vi "MC5e Check Unit is Unique.vi"(6 "index":i32, 7 "Mode":T7, 10 "Unit":T1={"Unit Fatigue Level"=enum."Not Fatigued", "Flying Unit"=FALSE, "Mounted Unit"=FALSE, "Defending from Stronghold"=FALSE, "Difficult Terrain Types"=[0, 1, 3, 6, 7], "Squads in Unit"=[], "Unit Info"={"Unit Name"="", "Unit Commander"="", "Morale Mod"=0, "BR Mod"=0, "Defense Mod"=0, "Speed Mod"=0, "Unit Notes"="", "Attack Mod"=0, "Unit Wins+ Losses-"=0, "Commander Charisma Bonus"=0}, "Range"=0, "BR"=0, "Speed"=0, "Morale"=0, "Current BR"=0, "Location"={"X coordinate"=0.0, "Y coordinate"=0.0}, "Capacity %"=0} {"Squads in Unit"."CR" items=["30", "29", "28", "27", "26", "25", "24", "23", "22", "21", "20", "19", "18", "17", "16", "15", "14", "13", "12", "11", "10", "9", "8", "7", "6", "5", "4", "3", "2", "1", "1/2", "1/4", "1/8"]}) -> (1 "Unit Name is Valid":bool, 2 "Unit Out (Duplicate)":T1={"Unit Fatigue Level"=enum."Not Fatigued", "Flying Unit"=FALSE, "Mounted Unit"=FALSE, "Defending from Stronghold"=FALSE, "Difficult Terrain Types"=[0, 1, 3, 6, 7], "Squads in Unit"=[], "Unit Info"={"Unit Name"="", "Unit Commander"="", "Morale Mod"=0, "BR Mod"=0, "Defense Mod"=0, "Speed Mod"=0, "Unit Notes"="", "Attack Mod"=0, "Unit Wins+ Losses-"=0, "Commander Charisma Bonus"=0}, "Range"=0, "BR"=0, "Speed"=0, "Morale"=0, "Current BR"=0, "Location"={"X coordinate"=0.0, "Y coordinate"=0.0}, "Capacity %"=0} {"Squads in Unit"."CR" items=["30", "29", "28", "27", "26", "25", "24", "23", "22", "21", "20", "19", "18", "17", "16", "15", "14", "13", "12", "11", "10", "9", "8", "7", "6", "5", "4", "3", "2", "1", "1/2", "1/4", "1/8"]}, 3 "OK Button Disabled?":T8(ring))   [LabVIEW 2020]
uses:
  MC5e Editor modes.ctl
  MC5e Unit.ctl
  MC5e Terrain types.ctl
  MC5e Squad_Info.ctl
  MC5e Size_Categories.ctl
  MC5e Unit Header.ctl
  Location.ctl
panel:
  # "Squads are restricted to one type of soldier (i.e  Archers) and all of the same level.\nIf you want mixed CR or mixed types, use multiple squads."
  # "Squads are restricted to one type of soldier (i.e  Archers) and all of the same level.\nIf you want mixed CR or mixed types, use multiple squads."
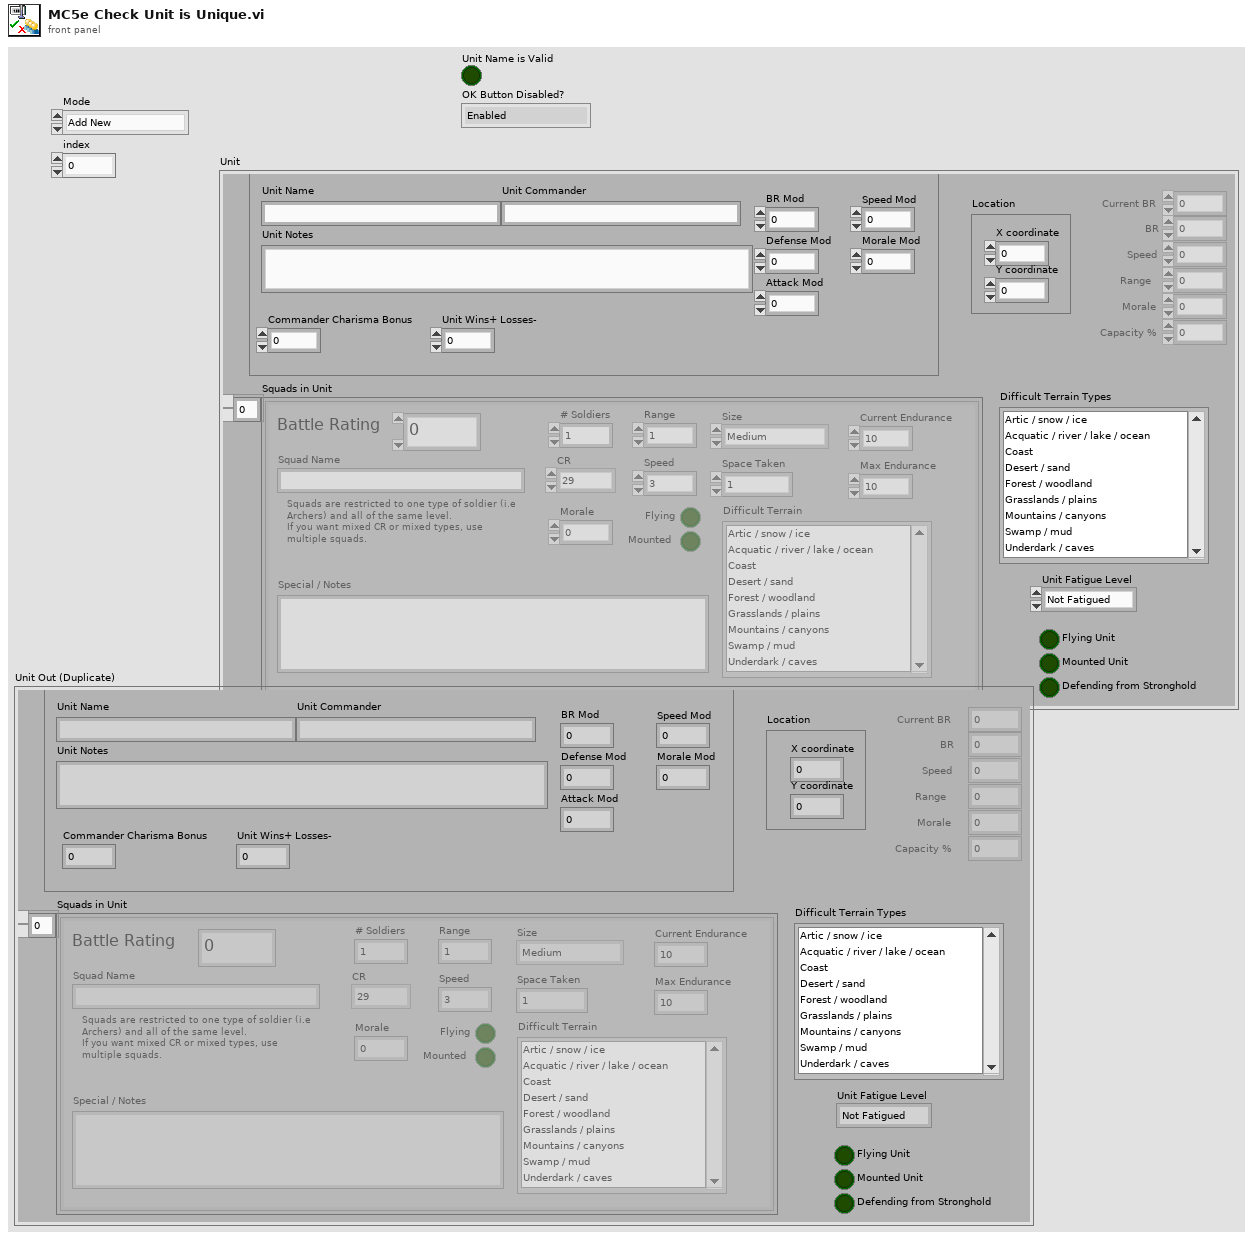
[diagram p1: front panel]
types:
  T1 = typedef "MC5e Unit.ctl" = cluster{"Unit Fatigue Level":enum16{"Not Fatigued", "Fatigued", "Seriously Fatigued"}, "Flying Unit":bool, "Mounted Unit":bool, "Defending from Stronghold":bool, "Difficult Terrain Types":T2, "Squads in Unit":T3[], "Unit Info":T5, "Range":i32, "BR":i32, "Speed":i32, "Morale":i32, "Current BR":i32, "Location":T6, "Capacity %":i32}
  T2 = typedef "MC5e Terrain types.ctl" = i32[]
  T3 = typedef "MC5e Squad_Info.ctl" = cluster{"Squad Name":string, "# Soldiers":u16, "Battle Rating":u16, "Flying":bool, "Mounted":bool, "Speed":u16, "Range":u16, "Morale":i32, "Max Endurance":u16, "Current Endurance":i32, "Size":T4, "Space Taken":u16, "Difficult Terrain":i32[], "CR":u16, "Special / Notes":string}
  T4 = typedef "MC5e Size_Categories.ctl" = enum16{"Tiny", "Small", "Medium", "Large", "Huge", "Gargantuan"}
  T5 = typedef "MC5e Unit Header.ctl" = cluster{"Unit Name":string, "Unit Commander":string, "Morale Mod":i32, "BR Mod":i32, "Defense Mod":i32, "Speed Mod":i32, "Unit Notes":string, "Attack Mod":i32, "Unit Wins+ Losses-":i32, "Commander Charisma Bonus":i32}
  T6 = typedef "Location.ctl" = cluster{"X coordinate":dbl, "Y coordinate":dbl}
  T7 = typedef "MC5e Editor modes.ctl" = enum16{"Add New", "Copy Selected", "Delete Selected", "Edit Selected"}
  T8 = enum8{"Enabled", "Disabled", "Disabled and Grayed Out"}
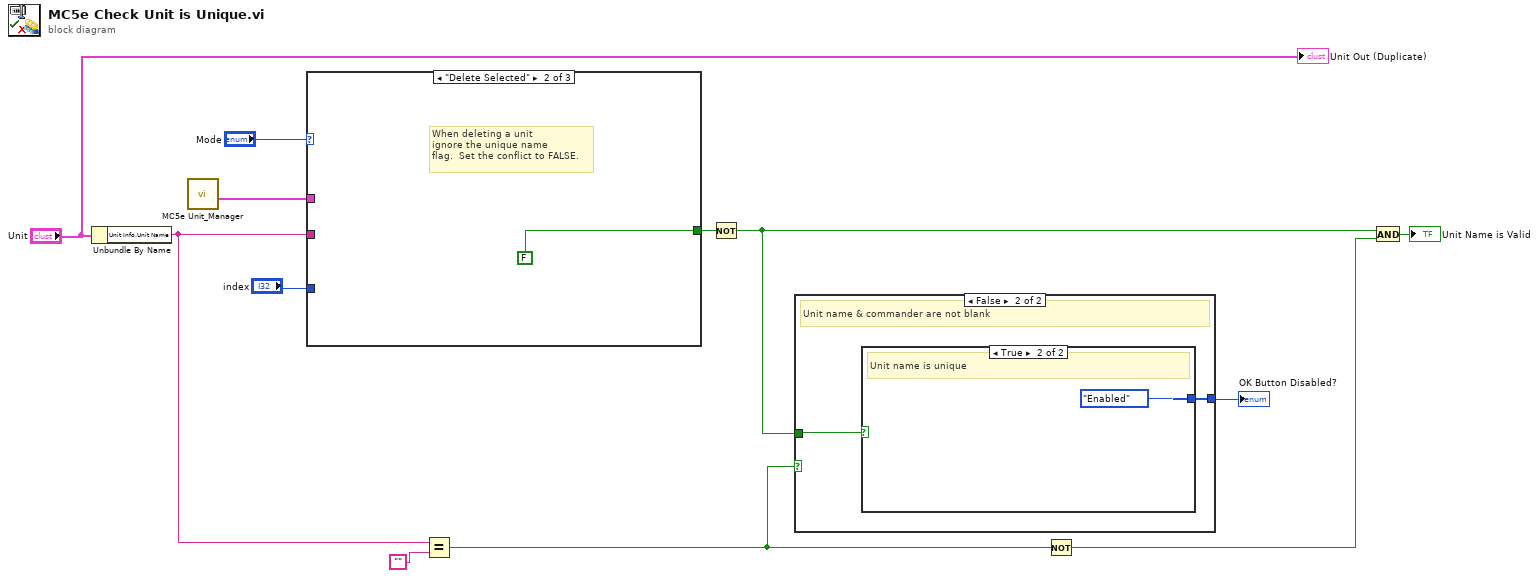
[diagram p0: block diagram]
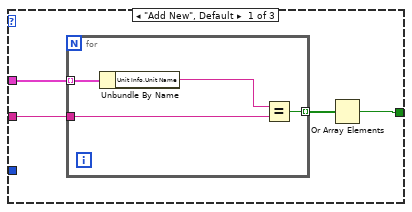
[diagram p2: hidden frame]
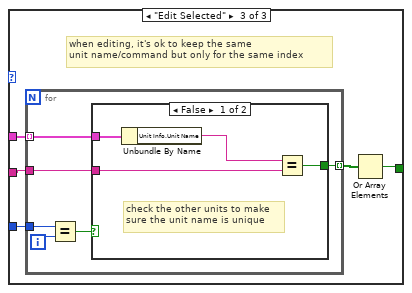
[diagram p3: hidden frame]
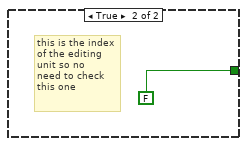
[diagram p4: hidden frame]
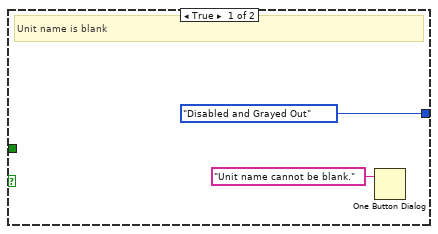
[diagram p5: hidden frame]
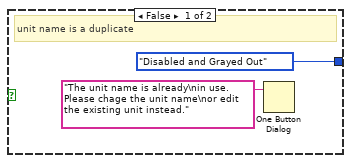
[diagram p6: hidden frame]
diagram:
  n1 = Unbundle By Name("Unit") -> ("Unit Info.Unit Name"=w2:string)
  n2 = call "MC5e Unit_Manager.vi"() -> ("All Units Out"=w6:T1[])  [unwired: 8 in, 3 out]
  n3 = case shown="\"Delete Selected\"" "Mode" {
    tunnel: [w15 FALSE w24] -> w12
    tunnel: w2 -> [w14 _ w25]
    tunnel: "index" -> [_ _ w23]
    tunnel: w6 -> [w13 _ w22]
    frame "Add New", Default {
      n4 = for {
        tunnel: [w20] -> w16 mode=indexing
        tunnel: w14 -> [w18]
        tunnel: w13 -> [w19] mode=indexing
        n5 = Unbundle By Name(w19) -> ("Unit Info.Unit Name"=w17:string)
        n6 = Equal?(x=w17, y=w18) -> (x = y?=w20:bool)
      }
      n7 = Or Array Elements(Boolean array=w16) -> (logical OR=w15:bool)
    }
    frame "Delete Selected" {
      # "When deleting a unit\nignore the unique name\nflag.  Set the conflict to FALSE."
    }
    frame "Edit Selected" {
      # "when editing, it's ok to keep the same\nunit name/command but only for the same index"
      n8 = for {
        tunnel: [w32] -> w26 mode=indexing
        tunnel: w25 -> [w31]
        tunnel: w23 -> [w29]
        tunnel: w22 -> [w27] mode=indexing
        i -> [w30]
        n9 = Equal?(x=w29, y=w30) -> (x = y?=w28:bool)
        n10 = case shown="False" w28 {
          tunnel: w27 -> [w36 _]
          tunnel: [w35 FALSE] -> w32
          tunnel: w31 -> [w33 _]
          frame False {
            # "check the other units to make\nsure the unit name is unique"
            n11 = Unbundle By Name(w36) -> ("Unit Info.Unit Name"=w34:string)
            n12 = Equal?(x=w34, y=w33) -> (x = y?=w35:bool)
          }
          frame True {
            # "this is the index\nof the editing\nunit so no \nneed to check\nthis one"
          }
        }
      }
      n13 = Or Array Elements(Boolean array=w26) -> (logical OR=w24:bool)
    }
  }
  n14 = Equal?(x=w2, y="") -> (x = y?=w5:bool)
  n15 = Not(x=w12) -> (.not. x?=w4:bool)
  n16 = case shown="False" w5 {
    tunnel: w4 -> [_ w41]
    tunnel: [T8."Disabled and Grayed Out" ("Disabled") w40] -> w11
    frame True {
      # "Unit name is blank"
      n17 = One Button Dialog(message="Unit name cannot be blank.") -> ()  [unwired: 1 in, 1 out]
    }
    frame False {
      # "Unit name & commander are not blank"
      n18 = case shown="True" w41 {
        tunnel: [T8."Disabled and Grayed Out" ("Disabled") T8."Enabled" ("Disabled")] -> w40
        frame False {
          # "unit name is a duplicate"
          n19 = One Button Dialog(message="The unit name is already\nin use.  Please chage the unit name\nor edit the existing unit instead.") -> ()  [unwired: 1 in, 1 out]
        }
        frame True {
          # "Unit name is unique"
        }
      }
    }
  }
  "OK Button Disabled?" <- w11
  n20 = Not(x=w5) -> (.not. x?=w1:bool)
  n21 = And(x=w4, y=w1) -> (x .and. y?=→"Unit Name is Valid":bool)
  "Unit Out (Duplicate)" <- "Unit"
